vi "ex3.vi"() -> ()   [LabVIEW 2022 SP3]
panel:
  out "concatenated string":string
  out "Date of birth":string
  in  "month":string
  in  "year":string
  in  "day":string
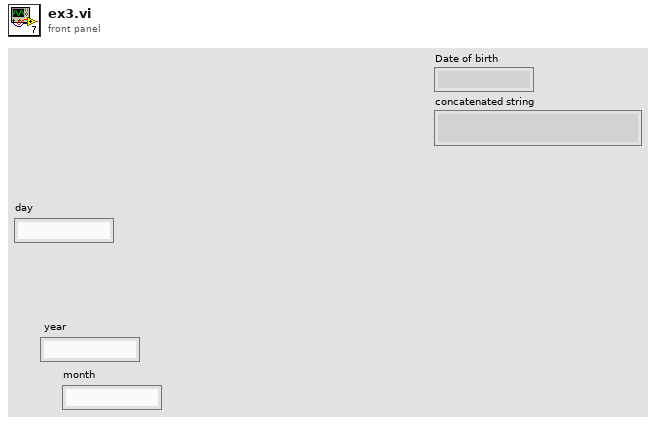
[diagram p1: front panel]
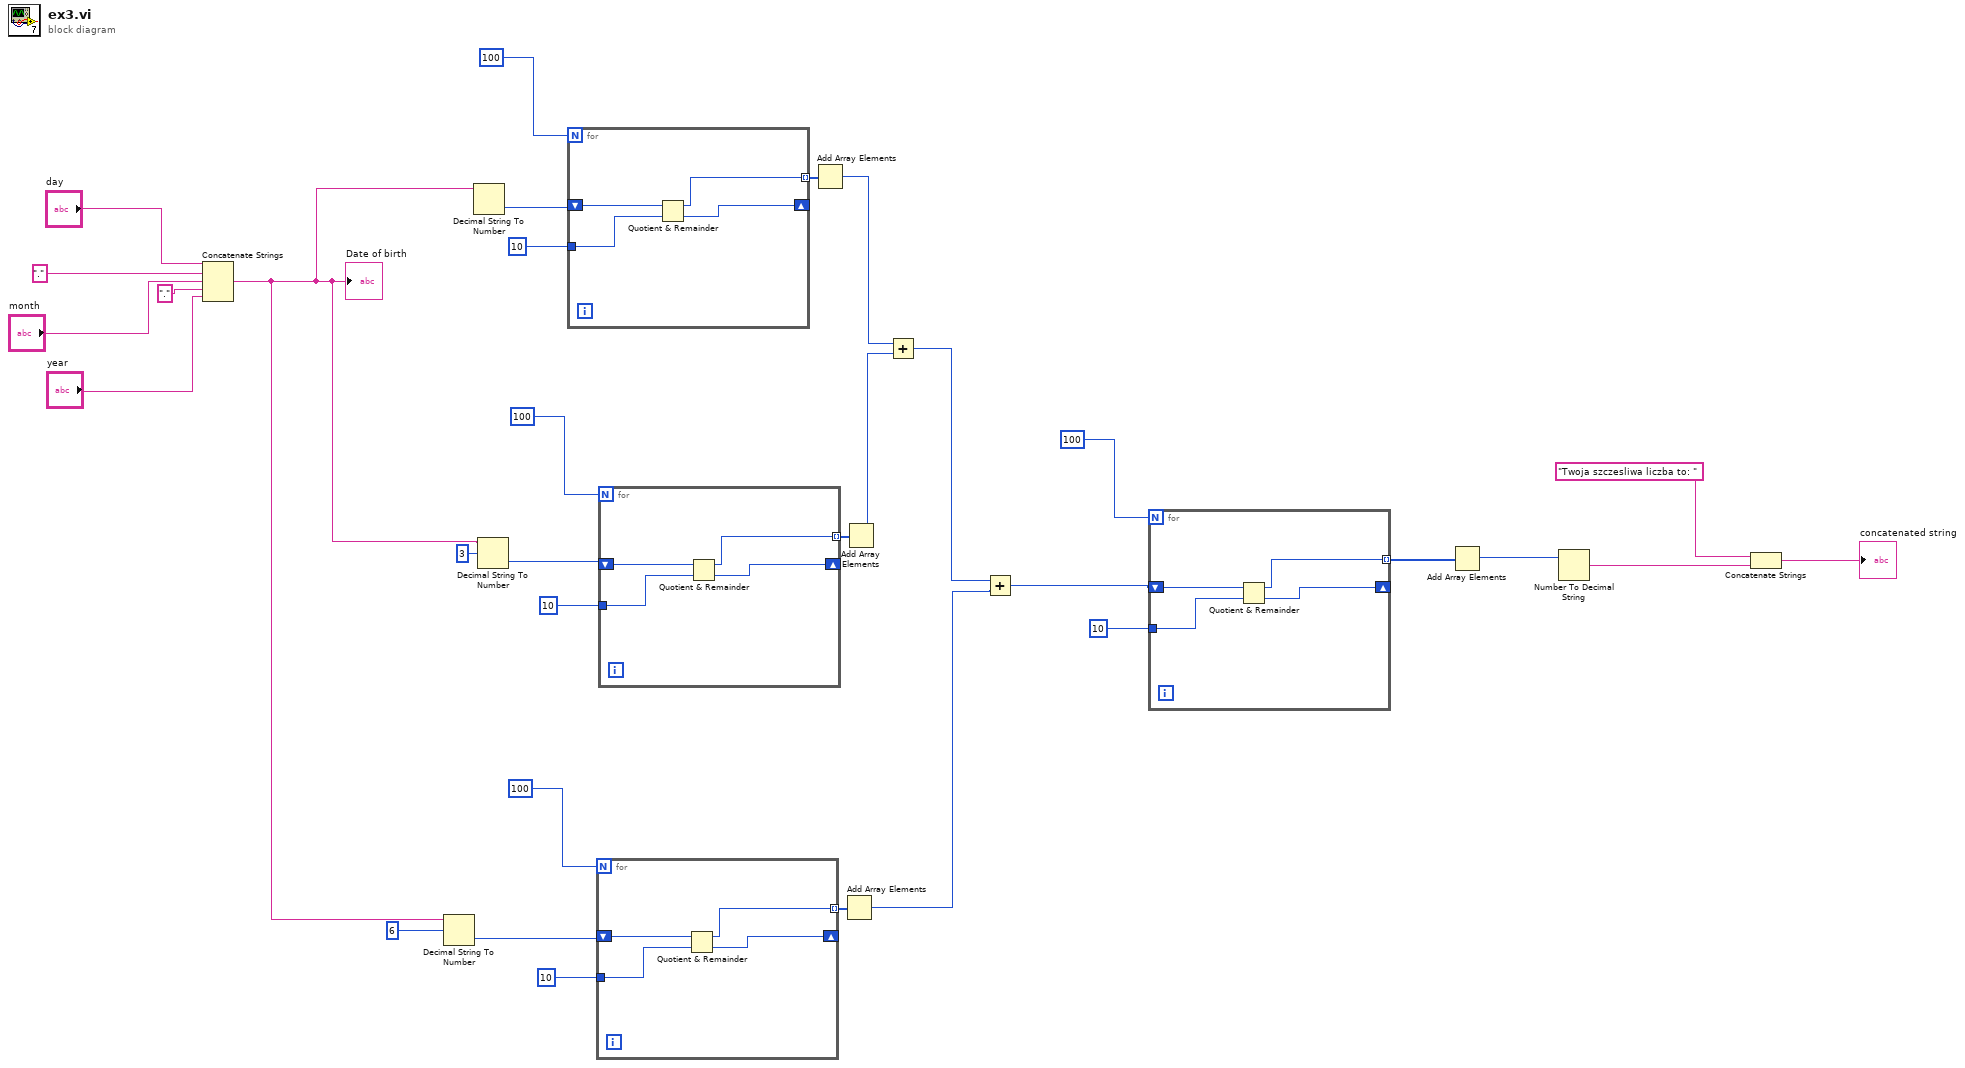
[diagram p0: block diagram]
diagram:
  n1 = Concatenate Strings("day", "." ("string"), "month", "." ("string"), "year") -> (w26:string)
  "Date of birth" <- w26
  n2 = Decimal String To Number(string=w26, offset=6) -> (number=w6:i32)  [unwired: 1 in, 1 out]
  n3 = Decimal String To Number(string=w26) -> (number=w15:i32)  [unwired: 2 in, 1 out]
  n4 = Decimal String To Number(string=w26, offset=3) -> (number=w10:i32)  [unwired: 1 in, 1 out]
  n5 = for {
    N: 100 -> [_]
    tunnel: 10 -> [w35]
    tunnel: [w34] -> w14 mode=indexing
    shift-right: [w33] -> _
    shift-left: w15 -> [w36]
    n6 = Quotient & Remainder(x=w36, y=w35) -> (x-y*floor(x/y)=w34:i32, floor(x/y)=w33:i32)
  }
  n7 = for {
    N: 100 -> [_]
    tunnel: 10 -> [w39]
    tunnel: [w38] -> w7 mode=indexing
    shift-right: [w37] -> _
    shift-left: w6 -> [w40]
    n8 = Quotient & Remainder(x=w40, y=w39) -> (x-y*floor(x/y)=w38:i32, floor(x/y)=w37:i32)
  }
  n9 = for {
    N: 100 -> [_]
    tunnel: 10 -> [w43]
    tunnel: [w42] -> w11 mode=indexing
    shift-right: [w41] -> _
    shift-left: w10 -> [w44]
    n10 = Quotient & Remainder(x=w44, y=w43) -> (x-y*floor(x/y)=w42:i32, floor(x/y)=w41:i32)
  }
  n11 = Add Array Elements(numeric array=w14) -> (sum=w5:i32)
  n12 = Add Array Elements(numeric array=w7) -> (sum=w2:i32)
  n13 = Add Array Elements(numeric array=w11) -> (sum=w4:i32)
  n14 = Add(x=w5, y=w4) -> (x+y=w3:i32)
  n15 = Add(x=w3, y=w2) -> (x+y=w1:i32)
  n16 = for {
    N: 100 -> [_]
    tunnel: 10 -> [w47]
    tunnel: [w46] -> w19 mode=indexing
    shift-right: [w45] -> _
    shift-left: w1 -> [w48]
    n17 = Quotient & Remainder(x=w48, y=w47) -> (x-y*floor(x/y)=w46:i32, floor(x/y)=w45:i32)
  }
  n18 = Add Array Elements(numeric array=w19) -> (sum=w18:i32)
  n19 = Number To Decimal String(number=w18) -> (decimal integer string=w23:string)  [unwired: 1 in]
  n20 = Concatenate Strings("Twoja szczesliwa liczba to: " ("string"), w23) -> (→"concatenated string":string)
